vi "H5D Write 1D Integer Call Lib.vi"(4 "xfer_plist_id":i32, 6 "file_space_id":i32, 7 "buf":u64[](array[numeric]), 8 "error in (no error)":errorcluster, 9 "mem_space_id":i32, 10 "mem_type_id":i32, 11 "dataset_id":i32) -> (0 "error out":errorcluster, 3 "dup dataset_id":i32)   [LabVIEW 2011]
uses:
  <instrlib>/Soft Front Panel File/hdf5dll.dll
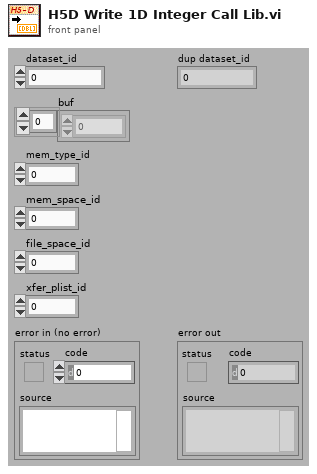
[diagram p1: front panel]
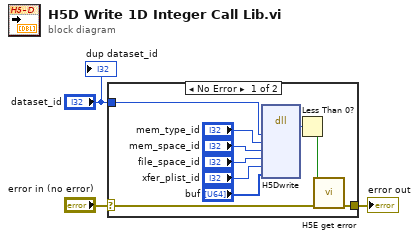
[diagram p0: block diagram]
diagram:
  n1 = case shown="No Error" "error in (no error)" {
    selector: "error in (no error)" -> [w5 w14]
    tunnel: "dataset_id" -> [w8 _]
    tunnel: [w4 w14] -> w2
    frame No Error {
      n2 = dll-call lib="D:/Program Files/National Instruments/LabVIEW 2011/instr.lib/Soft Front Panel File/hdf5dll.dll" fn="H5Dwrite"("dataset_id"=w8, "mem_type_id"="mem_type_id", "mem_space_id"="mem_space_id", "file_space_id"="file_space_id", "xfer_plist_id"="xfer_plist_id", "buf"="buf") -> ("return type"=w6:i32)  [unwired: 9 in, 2 out]
      n3 = Less Than 0?(x=w6) -> (x < 0?=w7:bool)
      n4 = call <instrlib>:"H5E get error.vi"("error in (no error)"=w5, "error?"=w7) -> ("error out"=w4:errorcluster)  [unwired: 9 in]
    }
    frame Error {
    }
  }
  "error out" <- w2
  "dup dataset_id" <- "dataset_id"
